vi "Access Level to String.vi"(1 "Access Level":T1=1 items=["Admin"=0, "User"=1, "Guest"=10]) -> (0 "String":string)   [LabVIEW 2016, in "UserPwd DB.lvlib" / "UserPwd DB Configuration.lvclass"]
uses:
  <userlib>/Common Components/UserPwd DB/UserPwd DB Config/UserPwd DB Configuration.lvclass
  <userlib>/Common Components/UserPwd DB/UserPwd DB Config/Access Level.ctl
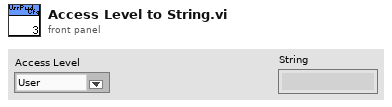
[diagram p1: front panel]
types:
  T1 = typedef "UserPwd DB.lvlib/UserPwd DB Configuration.lvclass/Access Level.ctl" = u16
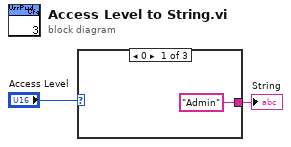
[diagram p0: block diagram]
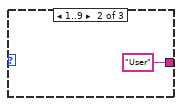
[diagram p2: hidden frame]
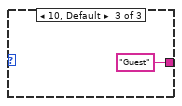
[diagram p3: hidden frame]
diagram:
  n1 = case shown="0" "Access Level" {
    tunnel: ["Admin" "User" "Guest"] -> w1
    frame 0 {
    }
    frame 1..9 {
    }
    frame 10, Default {
    }
  }
  "String" <- w1
